vi "Update Series.vi"(8 "error in (no error)":errorcluster, 10 "Series":T1={"Name"="", "Palette"=enum."None", "YAxisType"=enum."Primary", "XAxisType"=enum."Primary", "ChartType"=0, "Border"={"color"={"Color"=0, "alpha"=76}, "DashStyle"=enum."Solid", "Width"=2}, "Color"={"Color"=0, "alpha"=76}, "Marker"={"MarkerStyle"=enum."None", "Size"=0, "Step"=0, "Color"={"Color"=0, "alpha"=76}}} {"Marker"."Color"."alpha" scale=0.0..255.0; "Color"."alpha" scale=0.0..255.0; "Border"."color"."alpha" scale=0.0..255.0; "ChartType" items=["Point", "FastPoint", "Bubble", "Line", "Spline", "StepLine", "FastLine", "Bar", "StackedBar", "StackedBar100", "Column", "StackedColumn", "StackedColumn100", "Area", "SplineArea", "StackedArea", "StackedArea100", "Pie", "Doughnut", "Stock", "Candlestick", "Range", "SplineRange", "RangeBar", "RangeColumn", "Radar", "Polar", "ErrorBar", "BoxPlot", "Renko", "ThreeLineBreak", "Kagi", "PointAndFigure", "Funnel", "Pyramid"]}, 11 ".NET Refnum in":refnum<k24>) -> (0 "error out":errorcluster, 3 ".NET Refnum out":refnum<k24>)   [LabVIEW 2014, in "XMSChart.xctl"]
uses:
  XMSChart.xctl
  System.Windows.Forms.DataVisualization
  Controls/Series.ctl
  Controls/Border.ctl
  Controls/Color.ctl
  Controls/Marker.ctl
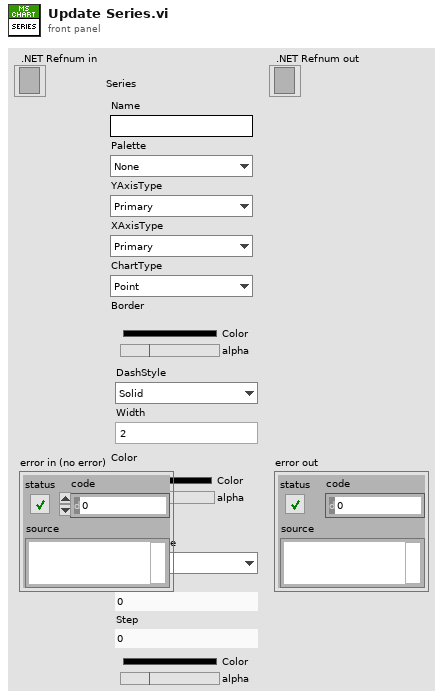
[diagram p1: front panel]
types:
  T1 = typedef "XMSChart.xctl/Series.ctl" = cluster{"Name":string, "Palette":enum16{"None", "Bright", "Grayscale", "Excel", "Light", "Pastel", "EarthTones", "SemiTransparent", "Berry", "Chocolate", "Fire", "SeaGreen", "BrightPastel"}, "YAxisType":enum16{"Primary", "Secondary"}, "XAxisType":enum16{"Primary", "Secondary"}, "ChartType":i32, "Border":T2, "Color":T3, "Marker":T4}
  T2 = typedef "XMSChart.xctl/Border.ctl" = cluster{"color":T3, "DashStyle":enum16{"NotSet", "Dash", "DashDot", "DashDotDot", "Dot", "Solid"}, "Width":i32}
  T3 = typedef "XMSChart.xctl/Color.ctl" = cluster{"Color":u32, "alpha":u8}
  T4 = typedef "XMSChart.xctl/Marker.ctl" = cluster{"MarkerStyle":enum16{"None", "Square", "Circle", "Diamond", "Triangle", "Cross", "Star4", "Star5", "Star6", "Star10"}, "Size":i32, "Step":i32, "Color":T3}
  T5 = enum16{"None", "Bright", "Grayscale", "Excel", "Light", "Pastel", "EarthTones", "SemiTransparent", "Berry", "Chocolate", "Fire", "SeaGreen", "BrightPastel"}
  T6 = enum16{"None", "Square", "Circle", "Diamond", "Triangle", "Cross", "Star4", "Star5", "Star6", "Star10"}
  T7 = enum16{"NotSet", "Dash", "DashDot", "DashDotDot", "Dot", "Solid"}
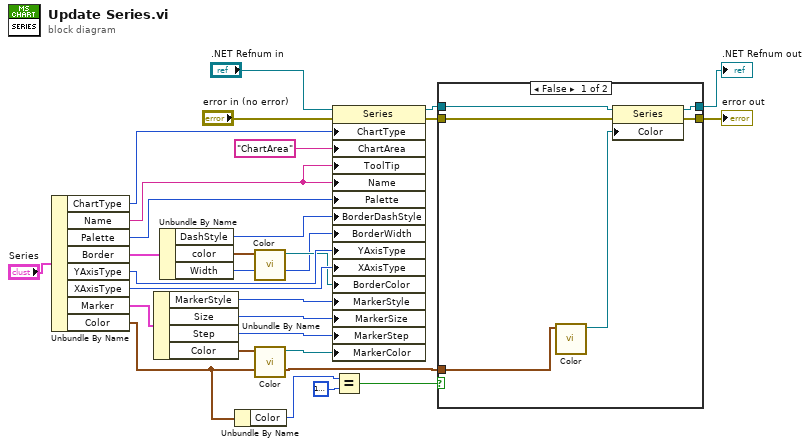
[diagram p0: block diagram]
diagram:
  n1 = Unbundle By Name("Series") -> ("ChartType"=w22:i32, "Name"=w19:string, "Palette"=w13:T5, "Border"=w7:T2, "YAxisType"=w15:enum16{"Primary", "Secondary"}, "XAxisType"=w16:enum16{"Primary", "Secondary"}, "Marker"=w14:T4, "Color"=w1:T3)
  n2 = Unbundle By Name(w14) -> ("MarkerStyle"=w17:T6, "Size"=w20:i32, "Step"=w21:i32, "Color"=w8:T3)
  n3 = Unbundle By Name(w7) -> ("DashStyle"=w6:T7, "color"=w5:T3, "Width"=w4:i32)
  n4 = Unbundle By Name(w1) -> ("Color"=w2:u32)
  n5 = call "Color.vi"("BGK Color"=w5) -> (".NET Refnum out"=w9:refnum<k24>)  [unwired: 10 in]
  n6 = call "Color.vi"("BGK Color"=w8) -> (".NET Refnum out"=w18:refnum<k24>)  [unwired: 10 in]
  n7 = property class="Series"(reference=".NET Refnum in", error in="error in (no error)", "ChartType"=w22, "ChartArea"="ChartArea", "ToolTip"=w19, "Name"=w19, "Palette"=w13, "BorderDashStyle"=w6, "BorderWidth"=w4, "YAxisType"=w15, "XAxisType"=w16, "BorderColor"=w9, "MarkerStyle"=w17, "MarkerSize"=w20, "MarkerStep"=w21, "MarkerColor"=w18) -> (reference out=w23:refnum<k24>, error out=w25:errorcluster)
  n8 = Equal?(x=w2, y=u32 16777216) -> (x = y?=w28:bool)
  n9 = case shown="False" w28 {
    tunnel: w1 -> [w29 _]
    tunnel: w23 -> [w34 w36]
    tunnel: [w33 w36] -> w24
    tunnel: w25 -> [w32 w35]
    tunnel: [w31 w35] -> w26
    frame False {
      n10 = call "Color.vi"("BGK Color"=w29) -> (".NET Refnum out"=w30:refnum<k24>)  [unwired: 10 in]
      n11 = property class="Series"(reference=w34, error in=w32, "Color"=w30) -> (reference out=w33:refnum<k24>, error out=w31:errorcluster)
    }
    frame True {
    }
  }
  "error out" <- w26
  ".NET Refnum out" <- w24
